vi "Keithley output configure.vi"(8 "error in (no error)":errorcluster, 10 "Keithley Output Configure":T1={"Sample Count (10)"=10, "Timeout (10000 ms)"=10000, "Compliance  Level (0.1)"=0.1, "Output Level (0)"=0.0, "Source Mode  (0: Voltage)"=0, "Output sequence"=0, "Output list"=[]} {"Source Mode  (0: Voltage)" items=["Voltage", "Current"]; "Timeout (10000 ms)" format="%#.6g"}, 11 "VISA resource name":refnum<visa-resource-name>) -> (0 "error out":errorcluster, 3 "VISA resource name out":refnum<visa-resource-name>)   [LabVIEW 2017]
uses:
  controls/Keithley input.ctl
  <instrlib>/Keithley 24XX/Keithley 24XX.lvlib
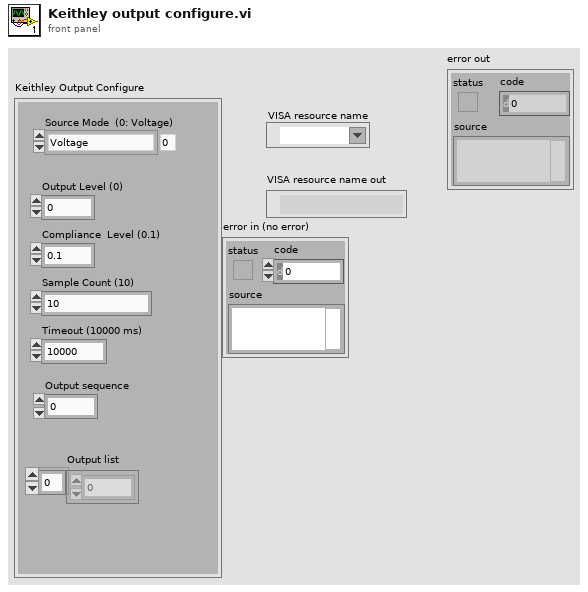
[diagram p1: front panel]
types:
  T1 = typedef "Keithley input.ctl" = cluster{"Sample Count (10)":i32, "Timeout (10000 ms)":i32, "Compliance  Level (0.1)":dbl, "Output Level (0)":dbl, "Source Mode  (0: Voltage)":u16, "Output sequence":i32, "Output list":dbl[]}
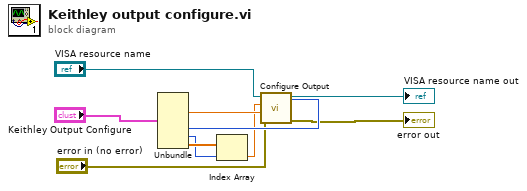
[diagram p0: block diagram]
diagram:
  n1 = Unbundle("Keithley Output Configure") -> ("Compliance  Level (0.1)"=w9:dbl, "Source Mode  (0: Voltage)"=w8:u16, "Output sequence"=w4:i32, "Output list"=w5:dbl[])  [unwired: 3 out]
  n2 = Index Array(array=w5, index=w4) -> (element=w3:dbl)
  n3 = call <instrlib>:"Configure Output.vi"("Source Mode  (0: Voltage)"=w8, "error in (no error)"="error in (no error)", "Compliance  Level (0.1)"=w9, "Output Level (0)"=w3, "VISA resource name"="VISA resource name") -> ("error out"=→"error out":errorcluster, "VISA resource name out"=→"VISA resource name out":refnum<visa-resource-name>)  [unwired: 5 in]
